vi "FA_ConvertFromAgentConfig.vi"(8 "Error In":errorcluster, 11 "AgentConfig":T3) -> (0 "Error Out":errorcluster, 3 "Config":T1)   [LabVIEW 2014, in "FA_AgentConfig.lvlib"]
doc: "Coverts from AgentConfig Special Type control to FA_NativeType's Config control."
uses:
  FA_AgentConfig.lvlib
  FA_AgentConfig.ctl
  FA_NativeTypes API/source/VI Source/FA_Config.ctl
  FA_LocalStore API/source/VI Source/FA_LSSpecialTypes.ctl
  FA_LocalStore API/source/VI Source/FA_LocalStore.lvlib
  FA_NativeTypes API/source/VI Source/FA_NativeTypes.lvlib
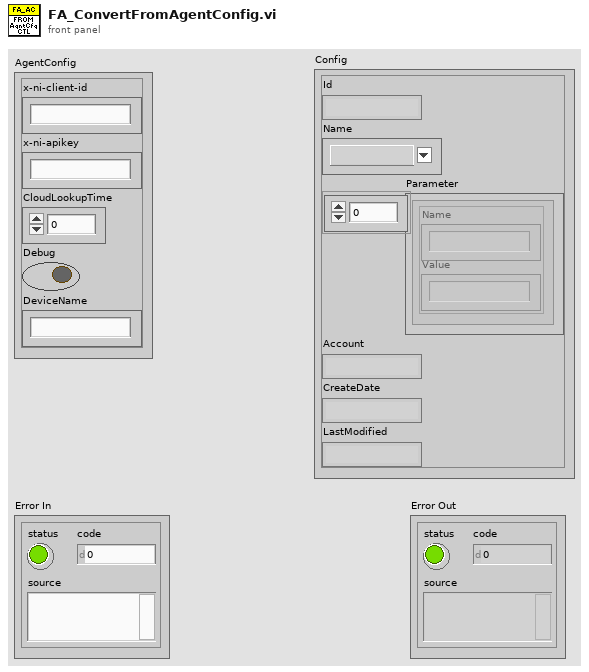
[diagram p1: front panel]
types:
  T1 = typedef "FA_NativeTypes.lvlib/FA_Config.ctl" = cluster{"Id":string, "Name":T2, "Parameter":cluster{"Name":string, "Value":string}[], "Account":string, "CreateDate":string, "LastModified":string}
  T2 = typedef "FA_LocalStore.lvlib/FA_LSSpecialTypes.ctl" = string
  T3 = typedef "FA_AgentConfig.lvlib/FA_AgentConfig.ctl" = cluster{"x-ni-client-id":string, "x-ni-apikey":string, "CloudLookupTime":u32, "Debug":bool, "DeviceName":string}
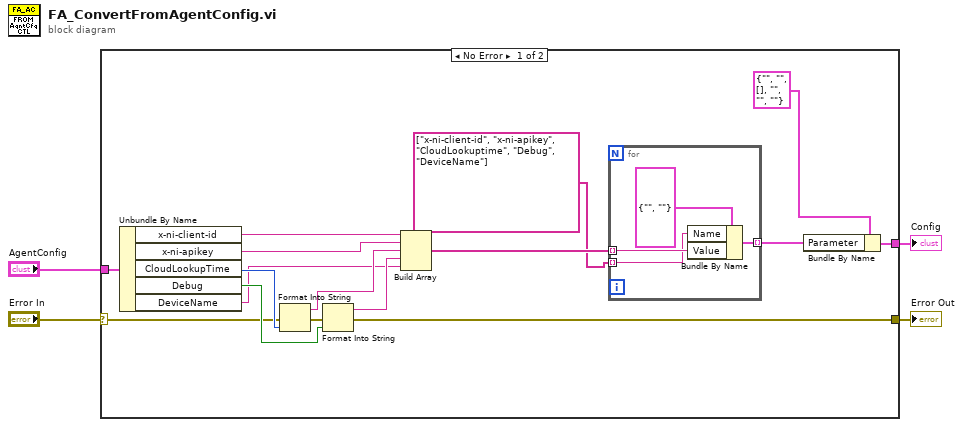
[diagram p0: block diagram]
diagram:
  n1 = case shown="No Error" "Error In" {
    selector: "Error In" -> [w8 w25]
    tunnel: [w6 w25] -> w1
    tunnel: "AgentConfig" -> [w20 _]
    tunnel: [w16 _] -> w2
    frame No Error {
      n2 = Unbundle By Name(w20) -> ("x-ni-client-id"=w15:string, "x-ni-apikey"=w14:string, "CloudLookupTime"=w19:u32, "Debug"=w18:bool, "DeviceName"=w9:string)
      n3 = Format Into String(error in=w8, w19) -> (resulting string=w13:string, error out=w7:errorcluster)  [unwired: 2 in]
      n4 = Format Into String(error in=w7, w18) -> (resulting string=w12:string, error out=w6:errorcluster)  [unwired: 2 in]
      n5 = Build Array(w15, w14, w13, w12, w9) -> (w11:string[])
      n6 = for {
        tunnel: w11 -> [w23] mode=indexing
        tunnel: string[] ["x-ni-client-id", "x-ni-apikey", "CloudLookuptime", "Debug", "DeviceName"] -> [w22] mode=indexing
        tunnel: [w21] -> w10 mode=indexing
        n7 = Bundle By Name(cluster=cluster{"Name":string, "Value":string} {"Name"="", "Value"=""} ("Parameter"), "Name"=w22, "Value"=w23) -> (w21:cluster{"Name":string, "Value":string})
      }
      n8 = Bundle By Name(cluster=T1 {"Id"="", "Name"="", "Parameter"=[], "Account"="", "CreateDate"="", "LastModified"=""} ("Config"), "Parameter"=w10) -> (w16:T1)
    }
    frame Error {
    }
  }
  "Config" <- w2
  "Error Out" <- w1
